vi "Charger_Status Refnum Prototype.vi"() -> ()   [LabVIEW 2010]
uses:
  Charger_Status Control.ctl
  Drivers/Charger Test Set/Charger_Input Control.ctl
  MICS_Input Control.ctl
panel:
  out "Charge Status":T1={"MICS ID"=4417, "VBAT"=nan, "ChargingState"="", "VBAT Slide"=3.5, "Status"="", "TemperatureLevel"=nan, "IPG_ReceivedLevel"=nan, "VBAT Target"=nan, "Charger Setpoint"=nan, "Index"=0, "Ready"=FALSE, "Charger Inputs"={"address"="COM17", "position"=0, "setpoint"=7500.0}, "MICS Inputs"={"address"="", "chan"=2, "ID"=0}} {"MICS Inputs"."ID" format="%06x"; "MICS Inputs"."chan" min=1 max=10 step=1; "Charger Inputs"."setpoint" min=0.0 max=20000.0 step=100.0; "Charger Inputs"."position" min=0 max=5 step=1; "MICS ID" format="%06x"; "VBAT Target" format="%.2f"; "VBAT Slide" scale=3.5..4.0 scale format="%.2f"; "VBAT" format="%.2f"}
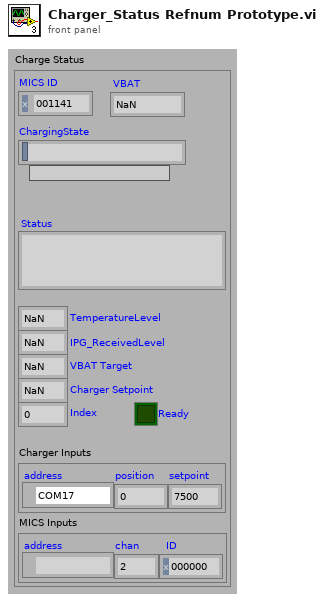
[diagram p1: front panel]
types:
  T1 = typedef "Charger_Status Control.ctl" = cluster{"MICS ID":u32, "VBAT":dbl, "ChargingState":string, "VBAT Slide":dbl, "Status":string, "TemperatureLevel":dbl, "IPG_ReceivedLevel":dbl, "VBAT Target":dbl, "Charger Setpoint":dbl, "Index":i32, "Ready":bool, "Charger Inputs":T2, "MICS Inputs":T3}
  T2 = typedef "Charger_Input Control.ctl" = cluster{"address":refnum<visa-resource-name>, "position":i32, "setpoint":dbl}
  T3 = typedef "MICS_Input Control.ctl" = cluster{"address":refnum<visa-resource-name>, "chan":u16, "ID":u32}
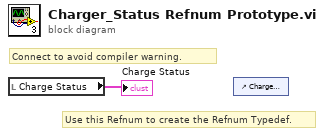
[diagram p0: block diagram]
diagram:
  # "Connect to avoid compiler warning."
  # "Use this Refnum to create the Refnum Typedef."
  n1 = local read "Charge Status"() -> (→"Charge Status":T1)
  n2 = control-ref of="Charge Status"() -> ()  [unwired: 1 out]
